vi "8BitsChar To 7bitsTokens.vi"(1 "Byte In":u16 format="%x") -> (0 "Byte Out":u32[](array[numeric]) format="%x")   [LabVIEW 2020]
doc: "The Firmata protocol reserves the 8th bit of every packet for its own operation. So any data that must be transferred\non the wire must be preprocessed. \n\nFor example a 8 bit data, is split over 2 bytes, the first byte will contain the least significant 7bits, and the last 8th \nbit is placed in the other byte (i.e 0xFF becomes [ 0xEF, 0x01 ])\n\nThe same logic can be applied for 16, 32,... bits data (0xFFAA becomes [ 0xEF, 0x01, 0x2A, 0x01 ])"
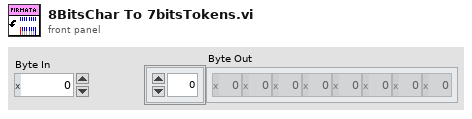
[diagram p1: front panel]
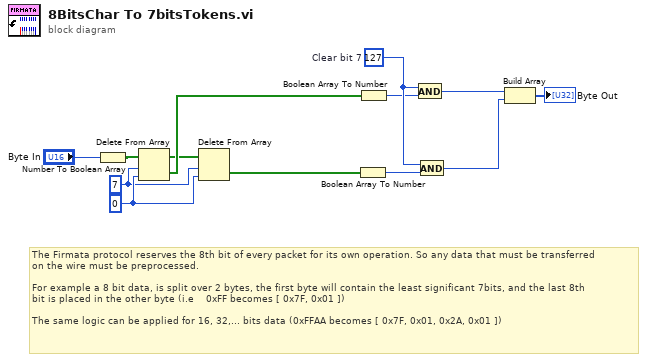
[diagram p0: block diagram]
diagram:
  w11 = u8 127  # Clear bit 7
  w5 = 7 ("length")
  w6 = 0 ("index")
  # "The Firmata protocol reserves the 8th bit of every packet for its own operation. So any data that must be transferred\non the wire must be preprocessed. \n\nFor example a 8 bit data, is split over 2 bytes, the first byte will contain the least significant 7bits, and the last 8th \nbit is placed in the other byte (i.e    0xFF becomes [ 0x7F, 0x01 ])\n\nThe same logic can be applied for 16, 32,... bits data (0xFFAA becomes [ 0x7F, 0x01, 0x2A, 0x01 ])"
  n1 = Number To Boolean Array(number="Byte In") -> (Boolean array=w13:bool[])
  n2 = Delete From Array(array=w13, length=w5, index=w6) -> (deleted portion=w7:bool[], array with subset deleted=w4:bool[])
  n3 = Delete From Array(array=w4, length=w5, index=w6) -> (deleted portion=w8:bool[])  [unwired: 1 out]
  n4 = Boolean Array To Number(Boolean array=w8) -> (number=w10:u32)
  n5 = Boolean Array To Number(Boolean array=w7) -> (number=w9:u32)
  n6 = And(x=w11, y=w9) -> (x .and. y?=w3:u32)
  n7 = And(x=w11, y=w10) -> (x .and. y?=w2:u32)
  n8 = Build Array(w3, w2) -> (→"Byte Out":u32[])
